vi "Read Branch Rate - Returns Default Value.vi"() -> ()   [LabVIEW 2017, in "Cobertura.Tests.lvlib" / "Package.lvlib"]
uses:
  Package.lvlib
  Cobertura/Package/Package.lvclass/Package.ctl
  Cobertura/Package/Read Branch Rate.vi
  <vilib>/PNR/Transparent Assertions/Transparent Assertions/Transparent Assertions.lvlib
  Cobertura/Package/Package.lvclass
panel:
  out "error out":errorcluster
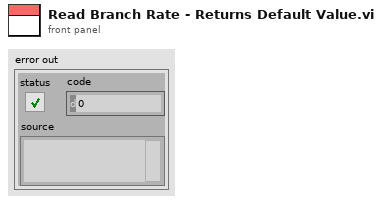
[diagram p1: front panel]
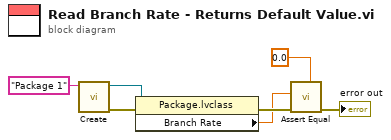
[diagram p0: block diagram]
diagram:
  n1 = call "Create.vi"("Name"="Package 1") -> ("error out"=w1:errorcluster, "Package"=w2:refnum<class "Package.lvclass">)  [unwired: 9 in]
  n2 = property class="Package.lvclass"(reference=w2, error in=w1) -> (error out=w7:errorcluster, "Branch Rate"=w5:dbl)  [unwired: 1 out]
  n3 = call <vilib>:"Assert Equal.vi"("Expected"=0.0 ("Branch Rate"), "error in (no error)"=w7, "Actual"=w5) -> ("error out"=→"error out":errorcluster)  [unwired: 8 in]
